vi "Unpack Panel Close.vi"(11 "PanelCloseMsg In":refnum<class "PanelCloseMsg.lvclass">) -> (1 "Discarded?":bool, 2 "Time":u32, 3 "Name":string)   [LabVIEW 2015, in "ActorAutoRegistration.lvlib" / "PanelCloseMsg.lvclass"]
uses:
  PanelCloseMsg.lvclass
  PanelCloseMsg.lvclass/PanelCloseMsg.ctl
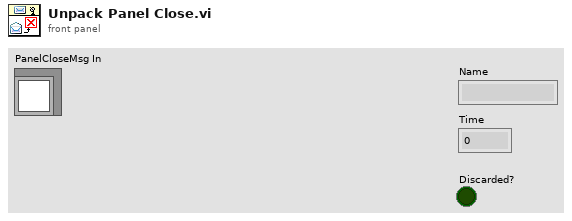
[diagram p1: front panel]
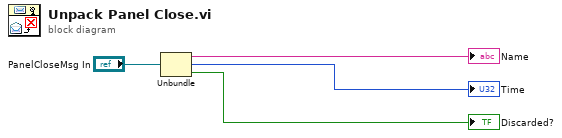
[diagram p0: block diagram]
diagram:
  n1 = Unbundle("PanelCloseMsg In") -> (→"Name":string, →"Time":u32, →"Discarded?":bool)
